vi "Block Correction.vi"() -> (0 "RL Dist":dbl, 1 "Block rad":dbl, 2 "Block Face":dbl, 3 "Close Range":dbl, 4 "Right Block":bool, 5 "Left Block":bool)   [LabVIEW 2018]
panel:
  out "theta":dbl
  out "Rad Array":dbl[](array[numeric])
  out "M Array":dbl[](array[numeric])
  out "Near Index":i32
  out "Y1":dbl
  out "Y2":dbl
  out "X2":dbl
  out "X1":dbl
  out "Array":dbl[](array[numeric])
  out "Index High":i32
  out "Index Low":i32
  out "Index Count":i32
  out "L Block Face":dbl
  out "L Block rad":dbl
  out "R Block Face":dbl
  out "R Block rad":dbl
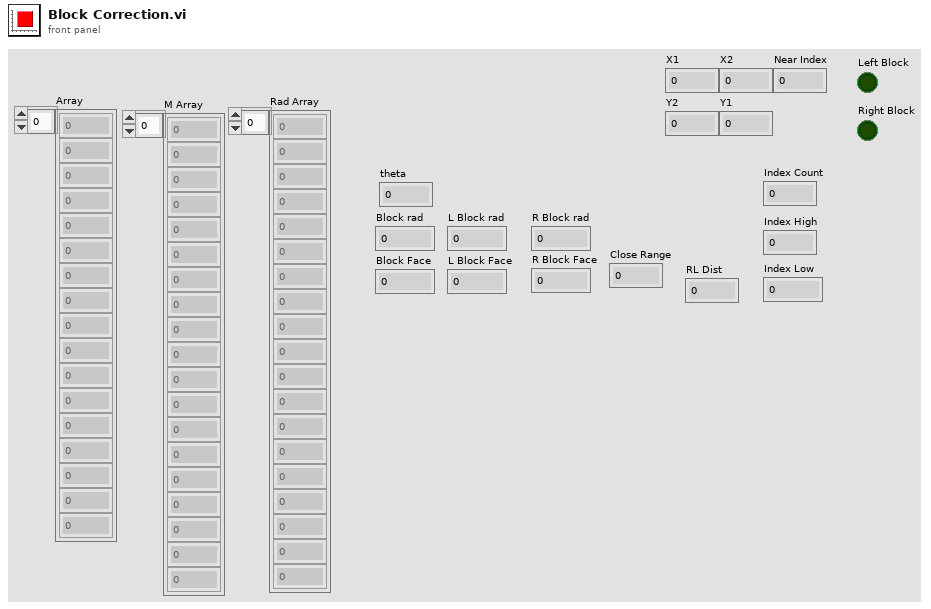
[diagram p1: front panel]
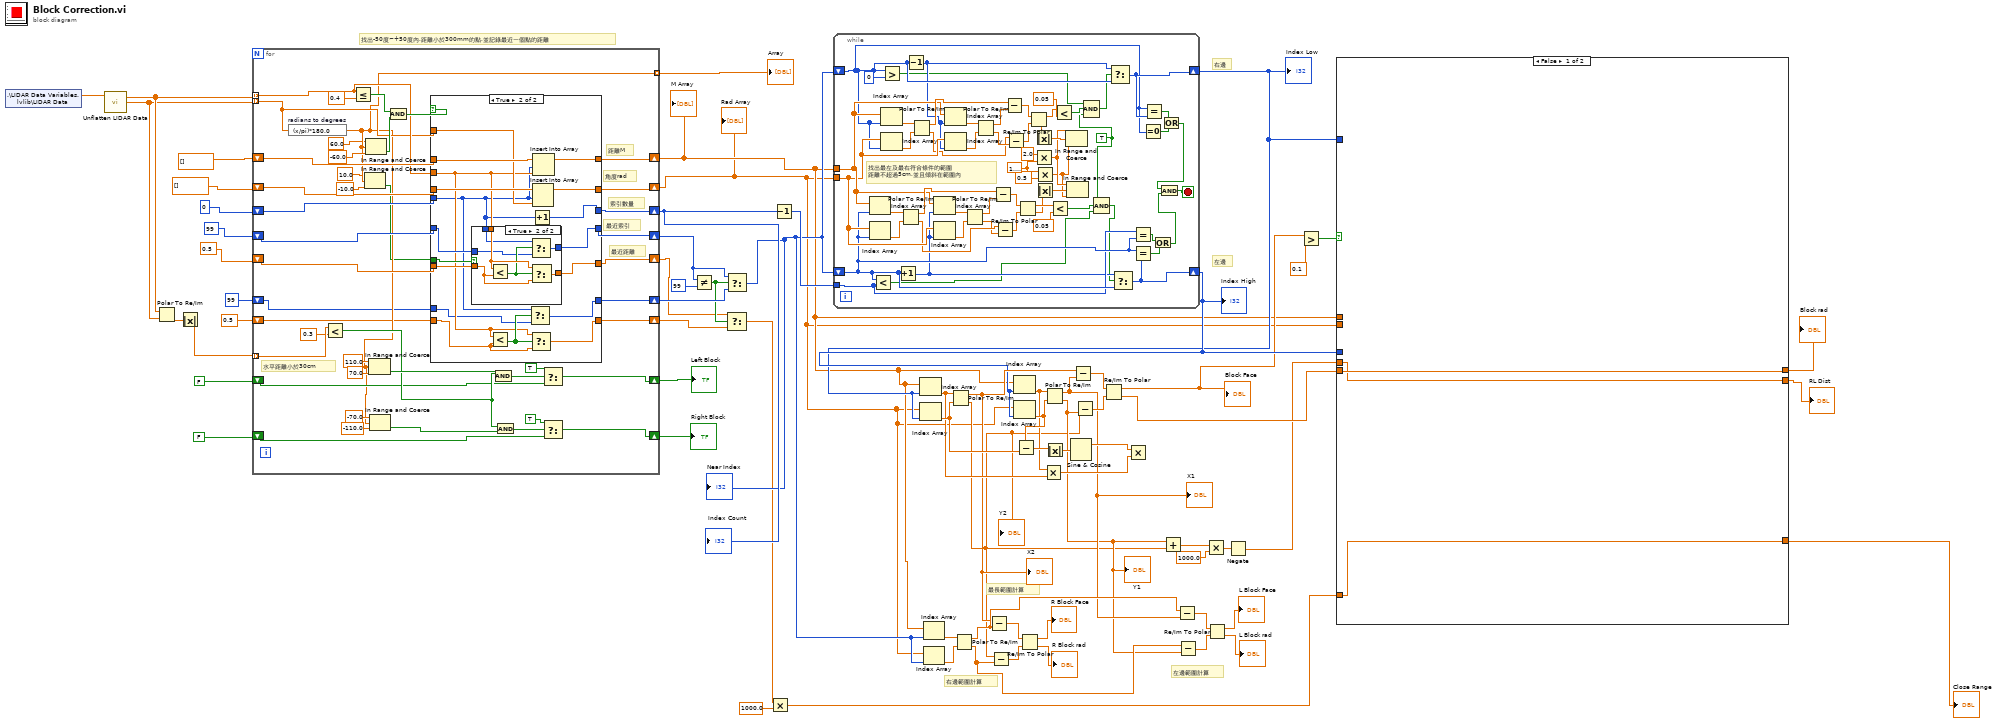
[diagram p0: block diagram]
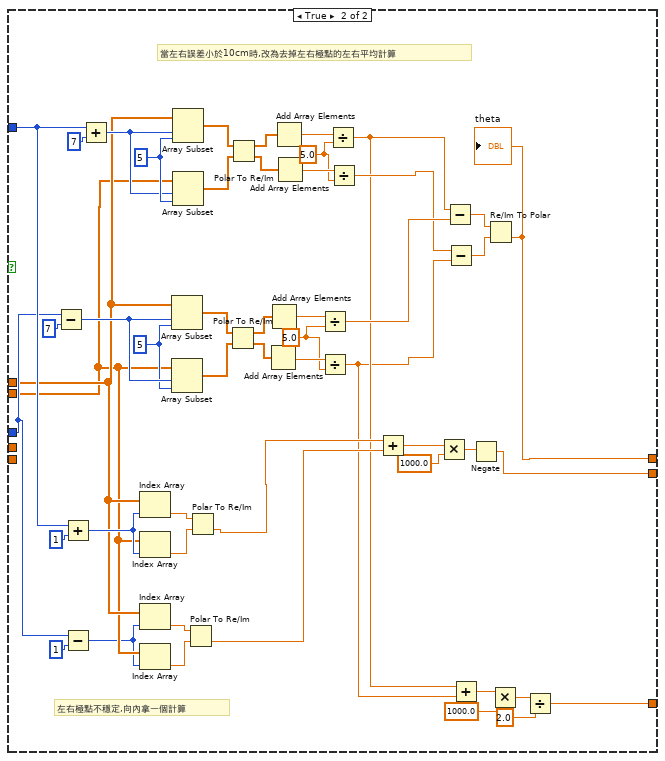
[diagram p2: hidden frame]
diagram:
  # "左邊範圍計算"
  # "右邊範圍計算"
  # "最長範圍計算"
  # "左邊"
  # "右邊"
  # "找出-50度~+50度內,距離小於300mm的點,並記錄最近一個點的距離"
  n1 = shared-variable ".\\LIDAR Data Variables.lvlib\\LIDAR Data"() -> (w63:dbl[])  [unwired: 1 in, 1 out]
  n2 = call "Unflatten LIDAR Data.vi"("Flat LIDAR Data"=w63) -> ("Bearing (rad)"=w59:dbl[], "Range (m)"=w60:dbl[])  [unwired: 7 in, 2 out]
  n3 = Polar To Re/Im(2:w59, 3:w60) -> (0:w58:dbl[])  [unwired: 1 out]
  n4 = Absolute Value(x=w58) -> (abs(x)=w57:dbl[])
  n5 = for {
    tunnel: w60 -> [w99] mode=indexing
    tunnel: w59 -> [w98] mode=indexing
    shift-right: [w106] -> w4
    shift-left: dbl[] [] -> [w109]
    shift-right: [w105] -> w3
    shift-left: dbl[] [] -> [w108]
    shift-right: [w100] -> w65
    shift-left: 0 -> [w107]
    shift-right: [w102] -> w16
    shift-left: 0.5 -> [w104]
    shift-right: [w101] -> w20
    shift-left: 99 -> [w103]
    tunnel: [w79] -> w61 mode=indexing
    tunnel: w57 -> [w97] mode=indexing
    shift-right: [w82] -> w54
    shift-left: FALSE -> [w86]
    shift-right: [w81] -> w53
    shift-left: FALSE -> [w85]
    shift-right: [w73] -> w18
    shift-left: 99 -> [w74]
    shift-right: [w72] -> w15
    shift-left: 0.5 -> [w71]
    # "水平距離小於30cm"
    # "索引數量"
    # "最近距離"
    # "最近索引"
    # "角度rad"
    # "距離M"
    n6 = expression code="(x/pi)*180.0" "radians to degrees"(w98) -> (w79:dbl)
    n7 = Less?(x=w97, y=0.3) -> (x < y?=w89:bool)
    n8 = Less Or Equal?(x=w99, y=0.4) -> (x <= y?=w112:bool)
    n9 = In Range and Coerce(upper limit=10.0, x=w79, lower limit=-10.0) -> (In Range?=w75:bool)  [unwired: 1 out]
    n10 = In Range and Coerce(upper limit=60.0, x=w79, lower limit=-60.0) -> (In Range?=w111:bool)  [unwired: 1 out]
    n11 = In Range and Coerce(upper limit=110.0, x=w79, lower limit=70.0) -> (In Range?=w90:bool)  [unwired: 1 out]
    n12 = In Range and Coerce(upper limit=-70.0, x=w79, lower limit=-110.0) -> (In Range?=w91:bool)  [unwired: 1 out]
    n13 = And(x=w112, y=w111) -> (x .and. y?=w110:bool)
    n14 = case shown="True" w110 {
      tunnel: w109 -> [w120 w138]
      tunnel: w108 -> [w119 w137]
      tunnel: w107 -> [w116 w125]
      tunnel: w99 -> [_ w126]
      tunnel: w98 -> [_ w136]
      tunnel: [w120 w135] -> w106
      tunnel: [w119 w134] -> w105
      tunnel: w104 -> [w118 w133]
      tunnel: w103 -> [w117 w129]
      tunnel: [w118 w132] -> w102
      tunnel: [w117 w131] -> w101
      tunnel: [w116 w130] -> w100
      tunnel: w75 -> [_ w128]
      tunnel: w74 -> [w115 w124]
      tunnel: [w115 w121] -> w73
      tunnel: [w114 w122] -> w72
      tunnel: w71 -> [w114 w123]
      frame False {
      }
      frame True {
        n15 = case shown="True" w128 {
          tunnel: w133 -> [w139 w147]
          tunnel: w126 -> [_ w146]
          tunnel: [w139 w145] -> w132
          tunnel: [w140 w143] -> w131
          tunnel: w125 -> [_ w142]
          tunnel: w129 -> [w140 w141]
          frame False {
          }
          frame True {
            n16 = Less?(x=w146, y=w147) -> (x < y?=w144:bool)
            n17 = Select(t=w142, s=w144, f=w141) -> (s? t:f=w143:i32)
            n18 = Select(t=w146, s=w144, f=w147) -> (s? t:f=w145:dbl)
          }
        }
        n19 = Less?(x=w126, y=w123) -> (x < y?=w127:bool)
        n20 = Select(t=w125, s=w127, f=w124) -> (s? t:f=w121:i32)
        n21 = Select(t=w126, s=w127, f=w123) -> (s? t:f=w122:dbl)
        n22 = Increment(x=w125) -> (x+1=w130:i32)
        n23 = Insert Into Array(array=w137, index=w125, new element=w136) -> (w134:dbl[])
        n24 = Insert Into Array(array=w138, index=w125, new element=w126) -> (w135:dbl[])
      }
    }
    n25 = And(x=w89, y=w90) -> (x .and. y?=w87:bool)
    n26 = And(x=w89, y=w91) -> (x .and. y?=w88:bool)
    n27 = Select(t=TRUE, s=w87, f=w86) -> (s? t:f=w82:bool)
    n28 = Select(t=TRUE, s=w88, f=w85) -> (s? t:f=w81:bool)
  }
  "Index Count" <- w65
  "Array" <- w61
  "Left Block" <- w54
  "Right Block" <- w53
  "M Array" <- w4
  "Rad Array" <- w3
  n29 = Not Equal?(x=w20, y=99) -> (x != y?=w17:bool)
  n30 = Select(t=w16, s=w17, f=w15) -> (s? t:f=w14:dbl)
  n31 = Select(t=w20, s=w17, f=w18) -> (s? t:f=w19:i32)
  "Near Index" <- w19
  n32 = Multiply(x=w14, y=1000.0) -> (x*y=w2:dbl)
  n33 = Decrement(x=w65) -> (x-1=w64:i32)
  n34 = while {
    tunnel: w4 -> [w183]
    tunnel: w3 -> [w182]
    shift-right: [w175] -> w13
    shift-left: w19 -> [w174]
    shift-right: [w177] -> w12
    shift-left: w19 -> [w176]
    tunnel: w64 -> [w173]
    stop <- w166 stop-if-true
    w148 = TRUE
    w160 = 1.5707963267948966
    # "找出最左及最右符合條件的範圍\n距離不超過5cm,並且傾斜在範圍內"
    n35 = Index Array(array=w183, index=w174) -> (element=w203:dbl)
    n36 = Index Array(array=w182, index=w174) -> (element=w202:dbl)
    n37 = Less?(x=w174, y=w173) -> (x < y?=w150:bool)
    n38 = Index Array(array=w183, index=w176) -> (element=w184:dbl)
    n39 = Index Array(array=w182, index=w176) -> (element=w185:dbl)
    n40 = Greater?(x=w176, y=0) -> (0:w154:bool)
    n41 = Increment(x=w174) -> (x+1=w162:i32)
    n42 = Polar To Re/Im(2:w202, 3:w203) -> (0:w181:dbl, 1:w199:dbl)
    n43 = Decrement(x=w176) -> (x-1=w163:i32)
    n44 = Polar To Re/Im(2:w185, 3:w184) -> (0:w178:dbl, 1:w188:dbl)
    n45 = Index Array(array=w183, index=w162) -> (element=w200:dbl)
    n46 = Index Array(array=w182, index=w162) -> (element=w201:dbl)
    n47 = Index Array(array=w183, index=w163) -> (element=w187:dbl)
    n48 = Index Array(array=w182, index=w163) -> (element=w186:dbl)
    n49 = Polar To Re/Im(2:w201, 3:w200) -> (0:w180:dbl, 1:w198:dbl)
    n50 = Polar To Re/Im(2:w186, 3:w187) -> (0:w179:dbl, 1:w189:dbl)
    n51 = Subtract(x=w199, y=w198) -> (x-y=w197:dbl)
    n52 = Subtract(x=w181, y=w180) -> (x-y=w196:dbl)
    n53 = Subtract(x=w188, y=w189) -> (x-y=w190:dbl)
    n54 = Subtract(x=w178, y=w179) -> (x-y=w191:dbl)
    n55 = Re/Im To Polar(2:w196, 3:w197) -> (0:w164:dbl, 1:w195:dbl)
    n56 = Re/Im To Polar(2:w191, 3:w190) -> (0:w165:dbl, 1:w192:dbl)
    n57 = Absolute Value(x=w165) -> (abs(x)=w161:dbl)
    n58 = Multiply(x=2.0, y=w160) -> (x*y=w156:dbl)
    n59 = Multiply(x=w160, y=0.5) -> (x*y=w155:dbl)
    n60 = Absolute Value(x=w164) -> (abs(x)=w157:dbl)
    n61 = Less?(x=w195, y=0.05) -> (x < y?=w151:bool)
    n62 = Less?(x=w192, y=0.05) -> (x < y?=w153:bool)
    n63 = In Range and Coerce(upper limit=w156, x=w161, lower limit=w155) -> ()  [unwired: 2 out]
    n64 = In Range and Coerce(upper limit=w156, x=w157, lower limit=w155) -> ()  [unwired: 2 out]
    n65 = Compound Arithmetic op=AND(w154, w153, w148) -> (w152:bool)
    n66 = Compound Arithmetic op=AND(w148, w151, w150) -> (w149:bool)
    n67 = Select(t=w163, s=w152, f=w176) -> (s? t:f=w177:i32)
    n68 = Select(t=w162, s=w149, f=w174) -> (s? t:f=w175:i32)
    n69 = Equal?(x=w173, y=w174) -> (x = y?=w170:bool)
    n70 = Equal?(x=w174, y=w175) -> (x = y?=w169:bool)
    n71 = Equal To 0?(x=w176) -> (x = 0?=w172:bool)
    n72 = Equal?(x=w176, y=w177) -> (x = y?=w171:bool)
    n73 = Or(x=w170, y=w169) -> (x .or. y?=w167:bool)
    n74 = Or(x=w171, y=w172) -> (x .or. y?=w168:bool)
    n75 = And(x=w168, y=w167) -> (x .and. y?=w166:bool)
  }
  "Index Low" <- w12
  "Index High" <- w13
  n76 = Index Array(array=w4, index=w12) -> (element=w33:dbl)
  n77 = Index Array(array=w3, index=w12) -> (element=w35:dbl)
  n78 = Index Array(array=w4, index=w19) -> (element=w49:dbl)
  n79 = Index Array(array=w3, index=w19) -> (element=w50:dbl)
  n80 = Polar To Re/Im(2:w35, 3:w33) -> (0:w25:dbl, 1:w27:dbl)
  "X2" <- w27
  "Y2" <- w25
  n81 = Polar To Re/Im(2:w50, 3:w49) -> (0:w39:dbl, 1:w40:dbl)
  n82 = Subtract(x=w27, y=w40) -> (x-y=w47:dbl)
  n83 = Subtract(x=w25, y=w39) -> (x-y=w48:dbl)
  n84 = Index Array(array=w4, index=w13) -> (element=w34:dbl)
  n85 = Index Array(array=w3, index=w13) -> (element=w36:dbl)
  n86 = Subtract(x=w36, y=w35) -> (x-y=w37:dbl)
  n87 = Re/Im To Polar(2:w48, 3:w47) -> (0:→"R Block rad":dbl, 1:→"R Block Face":dbl)
  n88 = Multiply(x=w34, y=w33) -> (x*y=w31:dbl)
  n89 = Polar To Re/Im(2:w36, 3:w34) -> (0:w26:dbl, 1:w30:dbl)
  "X1" <- w30
  "Y1" <- w26
  n90 = Absolute Value(x=w37) -> (abs(x)=w38:dbl)
  n91 = Sine & Cosine(0:w38) -> (1:w32:dbl)  [unwired: 1 out]
  n92 = Subtract(x=w27, y=w30) -> (x-y=w52:dbl)
  n93 = Subtract(x=w25, y=w26) -> (x-y=w51:dbl)
  n94 = Re/Im To Polar(2:w51, 3:w52) -> (0:w8:dbl, 1:w9:dbl)
  "Block Face" <- w9
  n95 = Multiply(x=w32, y=w31) -> ()  [unwired: 1 out]
  n96 = Add(x=w26, y=w25) -> (x+y=w28:dbl)
  n97 = Subtract(x=w40, y=w30) -> (x-y=w42:dbl)
  n98 = Subtract(x=w39, y=w26) -> (x-y=w41:dbl)
  n99 = Multiply(x=w28, y=1000.0) -> (x*y=w24:dbl)
  n100 = Re/Im To Polar(2:w41, 3:w42) -> (0:→"L Block rad":dbl, 1:→"L Block Face":dbl)
  n101 = Negate(x=w24) -> (-x=w6:dbl)
  n102 = Greater?(x=w9, y=0.1) -> (0:w11:bool)
  n103 = case shown="False" w11 {
    tunnel: w13 -> [_ w225]
    tunnel: w12 -> [_ w227]
    tunnel: w3 -> [_ w222]
    tunnel: w4 -> [_ w223]
    tunnel: w8 -> [w207 _]
    tunnel: [w207 w241] -> w7
    tunnel: w6 -> [w206 _]
    tunnel: [w206 w237] -> w5
    tunnel: w2 -> [w205 _]
    tunnel: [w205 w208] -> w1
    frame False {
    }
    frame True {
      w231 = 5.0 ("y")
      w234 = 5.0 ("y")
      w250 = 5 ("length")
      w255 = 5 ("length")
      # "左右極點不穩定,向內拿一個計算"
      # "當左右誤差小於10cm時,改為去掉左右極點的左右平均計算"
      n104 = Subtract(x=w225, y=7) -> (x-y=w256:i32)
      n105 = Add(x=w227, y=1) -> (x+y=w224:i32)
      n106 = Subtract(x=w225, y=1) -> (x-y=w221:i32)
      n107 = Add(x=w227, y=7) -> (x+y=w249:i32)
      n108 = Index Array(array=w223, index=w224) -> (element=w220:dbl)
      n109 = Index Array(array=w222, index=w224) -> (element=w219:dbl)
      n110 = Index Array(array=w223, index=w221) -> (element=w218:dbl)
      n111 = Index Array(array=w222, index=w221) -> (element=w217:dbl)
      n112 = Array Subset(array=w223, index=w256, length=w255) -> (w254:dbl[])
      n113 = Array Subset(array=w222, index=w256, length=w255) -> (w253:dbl[])
      n114 = Array Subset(array=w223, index=w249, length=w250) -> (w251:dbl[])
      n115 = Array Subset(array=w222, index=w249, length=w250) -> (w252:dbl[])
      n116 = Polar To Re/Im(2:w217, 3:w218) -> (0:w215:dbl)  [unwired: 1 out]
      n117 = Polar To Re/Im(2:w219, 3:w220) -> (0:w216:dbl)  [unwired: 1 out]
      n118 = Polar To Re/Im(2:w253, 3:w254) -> (0:w244:dbl[], 1:w245:dbl[])
      n119 = Polar To Re/Im(2:w252, 3:w251) -> (0:w246:dbl[], 1:w247:dbl[])
      n120 = Add Array Elements(numeric array=w244) -> (sum=w232:dbl)
      n121 = Add Array Elements(numeric array=w245) -> (sum=w233:dbl)
      n122 = Add Array Elements(numeric array=w247) -> (sum=w236:dbl)
      n123 = Add Array Elements(numeric array=w246) -> (sum=w235:dbl)
      n124 = Divide(x=w233, y=w231) -> (x/y=w230:dbl)
      n125 = Divide(x=w232, y=w231) -> (x/y=w213:dbl)
      n126 = Divide(x=w236, y=w234) -> (x/y=w214:dbl)
      n127 = Divide(x=w235, y=w234) -> (x/y=w229:dbl)
      n128 = Add(x=w216, y=w215) -> (x+y=w239:dbl)
      n129 = Multiply(x=w239, y=1000.0) -> (x*y=w240:dbl)
      n130 = Subtract(x=w214, y=w230) -> (x-y=w243:dbl)
      n131 = Subtract(x=w229, y=w213) -> (x-y=w242:dbl)
      n132 = Add(x=w214, y=w213) -> (x+y=w212:dbl)
      n133 = Negate(x=w240) -> (-x=w237:dbl)
      n134 = Re/Im To Polar(2:w242, 3:w243) -> (0:w241:dbl)  [unwired: 1 out]
      "theta" <- w241
      n135 = Multiply(x=w212, y=1000.0) -> (x*y=w210:dbl)
      n136 = Divide(x=w210, y=2.0) -> (x/y=w208:dbl)
    }
  }
  "Close Range" <- w1
  "RL Dist" <- w5
  "Block rad" <- w7
